vi "Scale Booleans.vi"(8 "error in (no error)":errorcluster, 11 "Data Scaling in":refnum<class "Data Scaling.lvclass">) -> (0 "error out":errorcluster, 3 "Data Scaling out":refnum<class "Data Scaling.lvclass">)   [LabVIEW 2020, in "Unit Tests.lvlib" / "Data Scaling.lvclass"]
uses:
  Data Scaling.lvclass
  Frames & Messages/TypeDefs/Scaling Information.ctl
  <vilib>/addons/_JKI Toolkits/Caraya/classes/Test/Test.lvclass
  <vilib>/addons/_JKI Toolkits/Caraya/classes/Assert/Assert.lvclass
  BCI-1553 API.lvlib
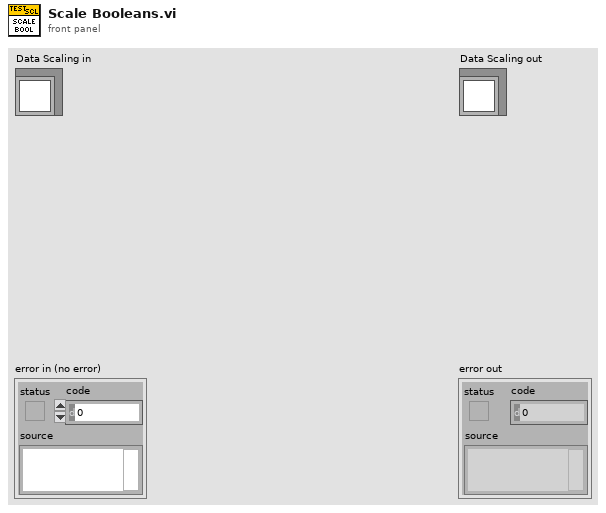
[diagram p1: front panel]
types:
  T1 = typedef "BCI-1553 API.lvlib/Scaling Information.ctl" = cluster{"Bit Offset":i32, "Bit Count":i32, "LSB Resolution":dbl, "2's Complement":bool, "Big Endian":bool, "Sign Bit":bool}
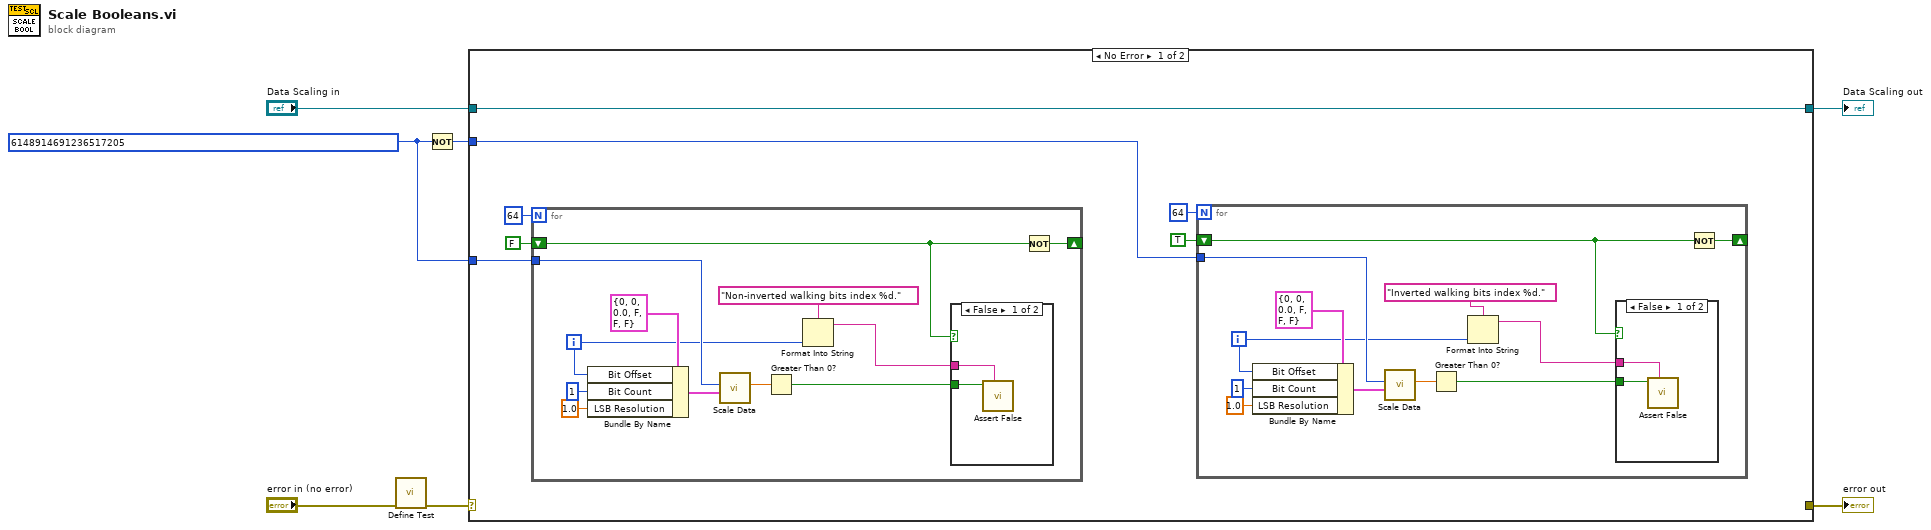
[diagram p0: block diagram]
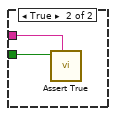
[diagram p2: hidden frame]
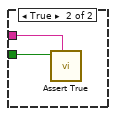
[diagram p3: hidden frame]
diagram:
  w2 = u64 6148914691236517205 ("Raw Value")
  n1 = call <vilib>:"Define Test.vi"("error in (no error)"="error in (no error)") -> ("error out"=w3:errorcluster)  [unwired: 9 in, 1 out]
  n2 = Not(x=w2) -> (.not. x?=w1:u64)
  n3 = case shown="No Error" w3 {
    selector: w3 -> [_ w48]
    tunnel: [_ w48] -> w7
    tunnel: [w14 w47] -> w5
    tunnel: "Data Scaling in" -> [w14 w47]
    tunnel: w2 -> [w11 _]
    tunnel: w1 -> [w10 _]
    frame No Error {
      n4 = for {
        N: 64 -> [_]
        shift-right: [w40] -> _
        shift-left: FALSE -> [w35]
        tunnel: w11 -> [w37]
        i -> [w32]
        n5 = Bundle By Name(cluster=T1 {"Bit Offset"=0, "Bit Count"=0, "LSB Resolution"=0.0, "2's Complement"=FALSE, "Big Endian"=FALSE, "Sign Bit"=FALSE} ("Scaling Info"), "Bit Offset"=w32, "Bit Count"=1, "LSB Resolution"=1.0) -> (w41:T1)
        n6 = call "Scale Data.vi"("Scaling Info"=w41, "Raw Value"=w37) -> ("Scaled Value"=w36:dbl)  [unwired: 8 in, 1 out]
        n7 = Greater Than 0?(x=w36) -> (x > 0?=w34:bool)
        n8 = Format Into String(format string="Non-inverted walking bits index %d.", w32) -> (resulting string=w31:string)  [unwired: 2 in, 1 out]
        n9 = case shown="False" w35 {
          tunnel: w34 -> [w44 w46]
          tunnel: w31 -> [w43 w45]
          frame False {
            n10 = call <vilib>:"Assert False.vi"("Label"=w43, "False?"=w44) -> ()  [unwired: 8 in, 2 out]
          }
          frame True {
            n11 = call <vilib>:"Assert True.vi"("Label"=w45, "True?"=w46) -> ()  [unwired: 8 in, 2 out]
          }
        }
        n12 = Not(x=w35) -> (.not. x?=w40:bool)
      }
      n13 = for {
        N: 64 -> [_]
        shift-right: [w24] -> _
        shift-left: TRUE -> [w19]
        tunnel: w10 -> [w21]
        i -> [w16]
        n14 = Bundle By Name(cluster=T1 {"Bit Offset"=0, "Bit Count"=0, "LSB Resolution"=0.0, "2's Complement"=FALSE, "Big Endian"=FALSE, "Sign Bit"=FALSE} ("Scaling Info"), "Bit Offset"=w16, "Bit Count"=1, "LSB Resolution"=1.0) -> (w25:T1)
        n15 = call "Scale Data.vi"("Scaling Info"=w25, "Raw Value"=w21) -> ("Scaled Value"=w20:dbl)  [unwired: 8 in, 1 out]
        n16 = Greater Than 0?(x=w20) -> (x > 0?=w18:bool)
        n17 = Format Into String(format string="Inverted walking bits index %d.", w16) -> (resulting string=w15:string)  [unwired: 2 in, 1 out]
        n18 = case shown="False" w19 {
          tunnel: w18 -> [w28 w30]
          tunnel: w15 -> [w27 w29]
          frame False {
            n19 = call <vilib>:"Assert False.vi"("Label"=w27, "False?"=w28) -> ()  [unwired: 8 in, 2 out]
          }
          frame True {
            n20 = call <vilib>:"Assert True.vi"("Label"=w29, "True?"=w30) -> ()  [unwired: 8 in, 2 out]
          }
        }
        n21 = Not(x=w19) -> (.not. x?=w24:bool)
      }
    }
    frame Error {
    }
  }
  "error out" <- w7
  "Data Scaling out" <- w5
